vi "process.vi"(8 "error in (no error)":errorcluster, 11 "Subscription in":refnum<class "Subscription.lvclass">) -> ()   [LabVIEW 2013, in "MQTT Base.lvlib" / "Subscription.lvclass"]
uses:
  Subscription.lvclass
  Subscription.lvclass/Subscription.ctl
  TopicFilter/TopicFilter.lvclass/TopicFilter.ctl
  TopicFilter/TopicFilter.lvclass
  <vilib>/LabVIEW Open Source Project/MQTT Control Packets/Control Packets/PUBLISH/PUBLISH.lvclass
panel:
  out "Topic Filter":string
  out "Numeric":i32
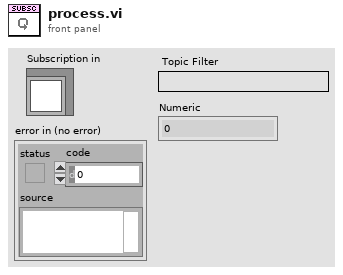
[diagram p1: front panel]
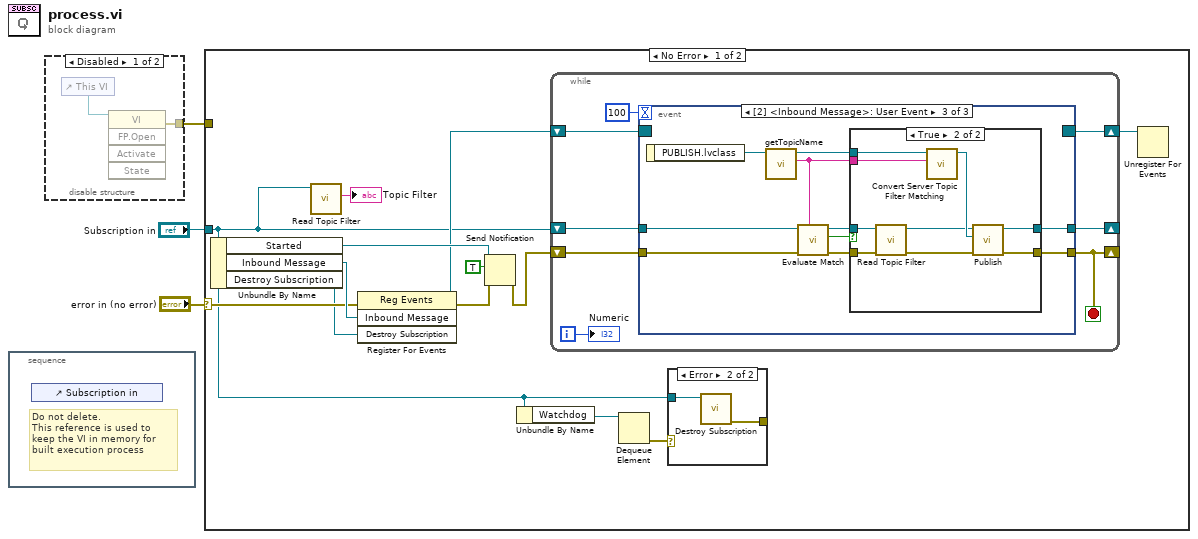
[diagram p0: block diagram]
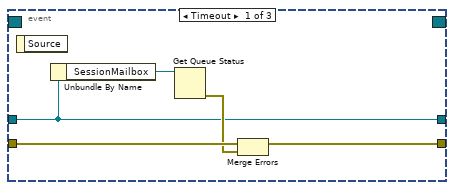
[diagram p4: hidden frame]
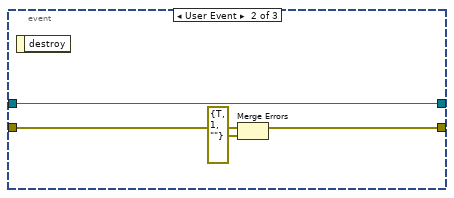
[diagram p5: hidden frame]
diagram:
  n1 = stacked-sequence {
    frame #0 {
      # "Do not delete.\nThis reference is used to keep the VI in memory for built execution process"
      n2 = control-ref of="Subscription in"() -> ()  [unwired: 1 out]
    }
  }
  n3 = disable-structure shown="Disabled" {
    disable-tunnel: [w4 _] -> w1
    frame Disabled {
      n4 = control-ref of="This VI"() -> (w5:refnum<vi>)
      n5 = invoke class="VI" method="FP.Open"(reference=w5) -> (error out=w4:errorcluster)  [unwired: 4 in, 4 out]
    }
    frame Enabled {
    }
  }
  n6 = case shown="No Error" "error in (no error)" {
    selector: "error in (no error)" -> [w14 _]
    tunnel: "Subscription in" -> [w6 _]
    tunnel: w1 -> [_ _]
    frame No Error {
      n7 = Unbundle By Name(w6) -> ("Started"=w16:refnum<notifier>, "Inbound Message"=w15:refnum<user-event>, "Destroy Subscription"=w9:refnum<user-event>)
      n8 = call "Read Topic Filter.vi"("Subscription in"=w6) -> ("Topic Filter"=→"Topic Filter":string)  [unwired: 7 in, 3 out]
      n9 = register-events(error in=w14, w15, w9) -> (reference out=w12:refnum<event-registration>, error out=w13:errorcluster)  [unwired: 1 in]
      n10 = Send Notification(notification=TRUE, notifier=w16, error in (no error)=w13) -> (error out=w17:errorcluster)  [unwired: 1 out]
      n11 = Unbundle By Name(w6) -> ("Watchdog"=w8:refnum<queue>)
      n12 = while {
        shift-right: [w23] -> _
        shift-left: w17 -> [w24]
        shift-right: [w26] -> w11
        shift-left: w12 -> [w27]
        shift-right: [w21] -> _
        shift-left: w6 -> [w25]
        i -> [w22]
        stop <- w23 stop-if-true
        n13 = event shown="[2] <Inbound Message>: User Event" {
          selector: w27 -> [_ _ _]
          dyn-events: [_ _ _] -> w26
          timeout: 100 -> [_ _ _]
          tunnel: w25 -> [w29 w35 w45]
          tunnel: w24 -> [w32 w37 w46]
          tunnel: [w30 w36 w47] -> w23
          tunnel: [w29 w35 w39] -> w21
          event Timeout {
            n14 = event-data() -> ()  [unwired: 1 in, 1 out]
            n15 = Unbundle By Name(w29) -> ("SessionMailbox"=w33:refnum<queue>)
            n16 = Get Queue Status(queue=w33) -> (error out=w31:errorcluster)  [unwired: 2 in, 7 out]
            n17 = Merge Errors(w32, w31) -> (w30:errorcluster)
          }
          event User Event {
            n18 = event-data() -> ()  [unwired: 1 in, 1 out]
            n19 = Merge Errors(w37, errorcluster {"status"=TRUE, "code"=1, "source"=""} ("error in")) -> (w36:errorcluster)
          }
          event User Event {
            n20 = event-data() -> ("PUBLISH.lvclass"=w44:refnum<class "PUBLISH.lvclass">)  [unwired: 1 in]
            n21 = call <vilib>:"getTopicName.vi"("PUBLISH in"=w44) -> ("Topic"=w38:string, "PUBLISH out"=w43:refnum<class "PUBLISH.lvclass">)  [unwired: 8 in, 1 out]
            n22 = call "Evaluate Match.vi"("Topic"=w38, "error in (no error)"=w46, "Subscription in"=w45) -> ("error out"=w40:errorcluster, "Matched"=w42:bool, "Subscription out"=w41:refnum<class "Subscription.lvclass">)  [unwired: 5 in, 1 out]
            n23 = case shown="True" w42 {
              tunnel: [w49 w58] -> w47
              tunnel: w40 -> [w49 w52]
              tunnel: w41 -> [w48 w54]
              tunnel: w43 -> [_ w56]
              tunnel: [w48 w57] -> w39
              tunnel: w38 -> [_ w50]
              frame False {
              }
              frame True {
                n24 = call "Read Topic Filter.vi"("error in (no error)"=w52, "Subscription in"=w54) -> ("error out"=w51:errorcluster, "Subscription out"=w53:refnum<class "Subscription.lvclass">)  [unwired: 6 in, 2 out]
                n25 = call <vilib>:"Convert Server Topic Filter Matching.vi"("Matching Topic Filter"=w50, "PUBLISH"=w56) -> ("Server PUBLISH"=w55:refnum<class "PUBLISH.lvclass">)  [unwired: 8 in, 1 out]
                n26 = call "Publish.vi"("error in (no error)"=w51, "PUBLISH"=w55, "Subscription in"=w53) -> ("error out"=w58:errorcluster, "Subscription out"=w57:refnum<class "Subscription.lvclass">)  [unwired: 7 in]
              }
            }
          }
        }
        "Numeric" <- w22
      }
      n27 = Dequeue Element(queue=w8) -> (error out=w7:errorcluster)  [unwired: 2 in, 3 out]
      n28 = case shown="Error" w7 {
        tunnel: w6 -> [_ w20]
        tunnel: [_ w19] -> _
        frame No Error {
        }
        frame Error {
          n29 = call "Destroy Subscription.vi"("Subscription in"=w20) -> ("error out"=w19:errorcluster)  [unwired: 9 in, 1 out]
        }
      }
      n30 = Unregister For Events(event registration refnum=w11) -> ()  [unwired: 1 in, 1 out]
    }
    frame Error {
    }
  }
